vi "Launch.vi"(9 "Alias":string, 10 "Actor":refnum<class "Actor.lvclass">) -> (0 "error out":errorcluster)   [LabVIEW 2021, in "jettl.lvlib" / "jettl.lvclass"]
uses:
  jettl.lvclass
  Actor/Actor/Actor.lvclass
  Launch jettl.vi
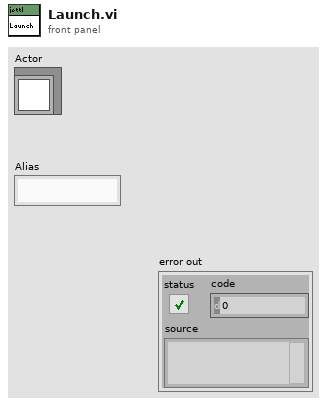
[diagram p1: front panel]
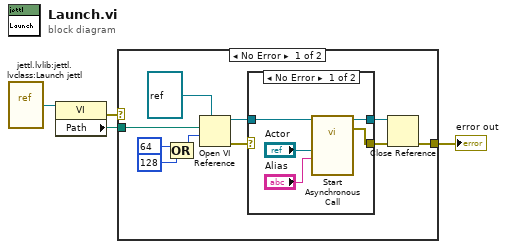
[diagram p0: block diagram]
diagram:
  n1 = vi-ref "jettl.lvlib:jettl.lvclass:Launch jettl.vi"() -> (w3:refnum<vi>)
  n2 = property class="VI"(reference=w3) -> (error out=w4:errorcluster, "Path"=w2:path)  [unwired: 1 in, 1 out]
  n3 = case shown="No Error" w4 {
    selector: w4 -> [_ w22]
    tunnel: [w12 w22] -> w1
    tunnel: w2 -> [w8 _]
    frame No Error {
      n4 = Compound Arithmetic op=OR(64 ("options: Multiple Clones,\n  Fire & Forget"), 128 ("options: Multiple Clones,\n  Fire & Forget")) -> (w10:i32)
      n5 = Open VI Reference(type specifier VI Refnum (for type only)=refnum<vi> refnum, vi path=w8, options=w10) -> (vi reference=w6:refnum<vi>, error out=w7:errorcluster)  [unwired: 3 in]
      n6 = case shown="No Error" w7 {
        selector: w7 -> [_ w21]
        tunnel: [w19 w20] -> w14
        tunnel: [w18 w21] -> w13
        tunnel: w6 -> [w17 w20]
        frame No Error {
          n7 = call-by-ref "Start Asynchronous Call"(reference=w17, "Alias"="Alias", "Actor"="Actor") -> (reference out=w19:refnum<vi>, error out=w18:errorcluster)  [unwired: 11 in]
        }
        frame Error {
        }
      }
      n8 = Close Reference(reference=w14, error in (no error)=w13) -> (error out=w12:errorcluster)
    }
    frame Error {
    }
  }
  "error out" <- w1
